vi "Open Btrfly Example.vi"() -> ()   [LabVIEW 2018]
uses:
  <vilib>/Rock Robotics/WPI/ThirdParty/Phoenix-LabVIEW/Motor Controller/Controls/CTRE_Phoenix_MotorControl_NeutralMode.ctl
  <vilib>/Rock Robotics/WPI/ThirdParty/REV Robotics/SPARK MAX/Typedef/Spark MAX Idle Mode.ctl
  <vilib>/Rock Robotics/WPI/SafetyOutput/WPI_SafetyOutputConfigMenu.ctl
  <vilib>/Rock Robotics/WPI/RobotDrive/WPI_RobotDriveOpen2MotorWithExistingMotors.vi
panel:
  in  "Error code":bool
  in  "Neutral Mode":enum16{"Coast", "Brake"}(ring)
  in  "secondsFromNeutralToFull":dbl format="%#_13g"
  in  "Cluster":T1
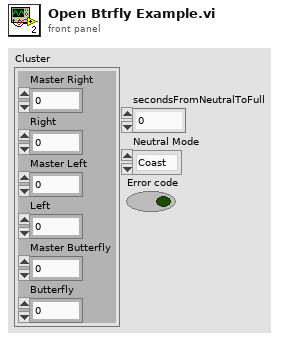
[diagram p1: front panel]
types:
  T1 = cluster{"Master Right":u8, "Right":u8, "Master Left":u8, "Left":u8, "Master Butterfly":u8, "Butterfly":u8}
  T2 = typedef "WPI_SafetyOutputConfigMenu.ctl" = enum16{"Enable", "Disable"}
  T3 = typedef "CTRE_Phoenix_MotorControl_NeutralMode.ctl" = enum8{"EEPROMSetting", "Override to Coast", "Override to Brake"}
  T4 = typedef "Spark MAX Idle Mode.ctl" = enum16{"Coast", "Brake"}
  T5 = typedef "WPI_MotorControlDeviceRef.ctl" = cluster{"DeviceStatus":errorcluster, "Type":T6, "PWM":cluster{"PWM Channel":T7, "DeadBand":T8}, "CAN":cluster{"Device Number":u8, "SetOutput VI Ref":variant, "GetOutput VI Ref":variant, "Enable VI Ref":variant, "Disable VI Ref":variant, "Data":variant}, "Invert":bool, "DIO PWM":cluster{"PWM \"Enable\" Channel":T7, "DIOChannel":T9, "PWM Rate":dbl}}
  T6 = typedef "WPI_MotorControlType.ctl" = enum16{"PWM", "CAN", "DIO PWM"}
  T7 = typedef "FPGA_DIOPWMChannel.ctl" = enum8{"PWM 0", "PWM 1", "PWM 2", "PWM 3", "PWM 4", "PWM 5", "PWM 6", "PWM 7", "PWM 8", "PWM 9", "PWM MXP 0", "PWM MXP 1", "PWM MXP 2", "PWM MXP 3", "PWM MXP 4", "PWM MXP 5", "PWM MXP 6", "PWM MXP 7", "PWM MXP 8", "PWM MXP 9", "Invalid"}
  T8 = typedef "WPI_PWMDeadband.ctl" = cluster{"Name":string, "maxPositivePwm":i32, "minPositivePwm":i32, "centerPwm":i32, "maxNegativePwm":i32, "minNegativePwm":i32, "angularRange":u16}
  T9 = typedef "FPGA_DIOChannel.ctl" = enum8{"DIO 0", "DIO 1", "DIO 2", "DIO 3", "DIO 4", "DIO 5", "DIO 6", "DIO 7", "DIO 8", "DIO 9", "DIO MXP 0", "DIO MXP 1", "DIO MXP 2", "DIO MXP 3", "DIO MXP 4", "DIO MXP 5", "DIO MXP 6", "DIO MXP 7", "DIO MXP 8", "DIO MXP 9", "DIO MXP 10", "DIO MXP 11", "DIO MXP 12", "DIO MXP 13", "DIO MXP 14", "DIO MXP 15", "SPI Port CS1", "SPI Port CS2", "SPI Port CS3", "SPI Port MISO", "SPI Port MOSI", "Invalid"}
  T10 = typedef "WPI_RobotDriveDevRef.ctl" = cluster{"DevStatus":errorcluster, "Motors[]":T5[], "Square Inputs":bool, "Max Output":dbl}
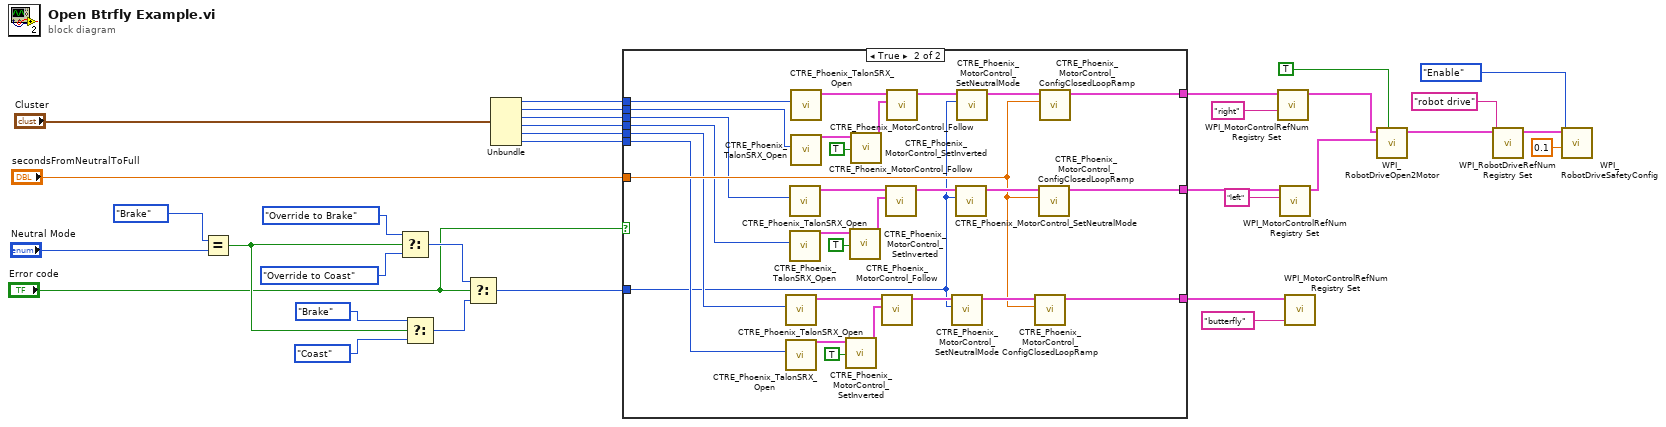
[diagram p0: block diagram]
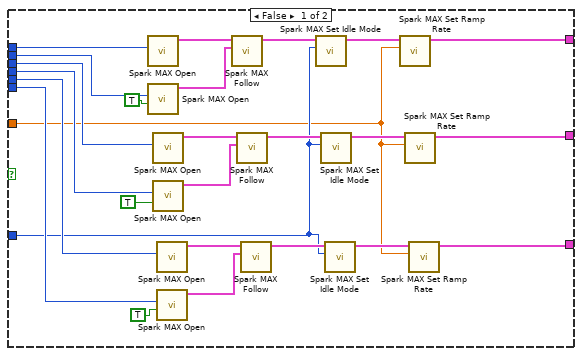
[diagram p2: hidden frame]
diagram:
  n1 = Equal?(x=enum16{"Coast", "Brake"}."Brake", y="Neutral Mode") -> (x = y?=w20:bool)
  n2 = Select(t=CTRE_Phoenix_MotorControl_NeutralMode."Override to Brake" ("Motor Control Neutral Mode"), s=w20, f=CTRE_Phoenix_MotorControl_NeutralMode."Override to Coast" ("Motor Control Neutral Mode")) -> (s? t:f=w21:T3)
  n3 = Select(t=Spark_MAX_Idle_Mode."Brake" ("Idle Mode"), s=w20, f=Spark_MAX_Idle_Mode."Coast" ("Idle Mode")) -> (s? t:f=w17:T4)
  n4 = Select(t=w21, s="Error code", f=w17) -> (s? t:f=w16:u16)
  n5 = Unbundle("Cluster") -> ("Master Right"=w31:u8, "Right"=w30:u8, "Master Left"=w29:u8, "Left"=w28:u8, "Master Butterfly"=w27:u8, "Butterfly"=w26:u8)
  n6 = case shown="True" "Error code" {
    tunnel: "secondsFromNeutralToFull" -> [w37 w70]
    tunnel: w31 -> [w46 w69]
    tunnel: w30 -> [w45 w68]
    tunnel: w29 -> [w44 w67]
    tunnel: w28 -> [w43 w66]
    tunnel: w27 -> [w42 w65]
    tunnel: w26 -> [w39 w64]
    tunnel: w16 -> [w38 w63]
    tunnel: [w36 w62] -> w14
    tunnel: [w35 w61] -> w13
    tunnel: [w34 w60] -> w12
    frame False {
      n7 = call <vilib>:"Spark MAX Open.vi"("Device Number"=w46) -> ("MotorControlDeviceRef"=w56:T5)  [unwired: 9 in, 1 out]
      n8 = call <vilib>:"Spark MAX Open.vi"("Invert"=TRUE, "Device Number"=w45) -> ("MotorControlDeviceRef"=w57:T5)  [unwired: 8 in, 1 out]
      n9 = call <vilib>:"Spark MAX Open.vi"("Device Number"=w44) -> ("MotorControlDeviceRef"=w54:T5)  [unwired: 9 in, 1 out]
      n10 = call <vilib>:"Spark MAX Open.vi"("Invert"=TRUE, "Device Number"=w43) -> ("MotorControlDeviceRef"=w53:T5)  [unwired: 8 in, 1 out]
      n11 = call <vilib>:"Spark MAX Open.vi"("Device Number"=w42) -> ("MotorControlDeviceRef"=w47:T5)  [unwired: 9 in, 1 out]
      n12 = call <vilib>:"Spark MAX Open.vi"("Invert"=TRUE, "Device Number"=w39) -> ("MotorControlDeviceRef"=w48:T5)  [unwired: 8 in, 1 out]
      n13 = call <vilib>:"Spark MAX Follow.vi"("Master Controller"=w57, "MotorControlDeviceRef"=w56) -> ("MotorControlDeviceRef"=w58:T5)  [unwired: 8 in, 1 out]
      n14 = call <vilib>:"Spark MAX Follow.vi"("Master Controller"=w53, "MotorControlDeviceRef"=w54) -> ("MotorControlDeviceRef"=w52:T5)  [unwired: 8 in, 1 out]
      n15 = call <vilib>:"Spark MAX Follow.vi"("Master Controller"=w48, "MotorControlDeviceRef"=w47) -> ("MotorControlDeviceRef"=w49:T5)  [unwired: 8 in, 1 out]
      n16 = call <vilib>:"Spark MAX Set Idle Mode.vi"("Idle Mode"=w38, "MotorControlDeviceRef in"=w58) -> ("MotorControlDeviceRef out"=w59:T5)  [unwired: 8 in, 1 out]
      n17 = call <vilib>:"Spark MAX Set Idle Mode.vi"("Idle Mode"=w38, "MotorControlDeviceRef in"=w52) -> ("MotorControlDeviceRef out"=w51:T5)  [unwired: 8 in, 1 out]
      n18 = call <vilib>:"Spark MAX Set Idle Mode.vi"("Idle Mode"=w38, "MotorControlDeviceRef in"=w49) -> ("MotorControlDeviceRef out"=w50:T5)  [unwired: 8 in, 1 out]
      n19 = call <vilib>:"Spark MAX Set Ramp Rate.vi"("Seconds from neutral to full (0)"=w37, "MotorControlDeviceRef in"=w59) -> ("MotorControlDeviceRef"=w36:T5)  [unwired: 8 in, 1 out]
      n20 = call <vilib>:"Spark MAX Set Ramp Rate.vi"("Seconds from neutral to full (0)"=w37, "MotorControlDeviceRef in"=w51) -> ("MotorControlDeviceRef"=w35:T5)  [unwired: 8 in, 1 out]
      n21 = call <vilib>:"Spark MAX Set Ramp Rate.vi"("Seconds from neutral to full (0)"=w37, "MotorControlDeviceRef in"=w50) -> ("MotorControlDeviceRef"=w34:T5)  [unwired: 8 in, 1 out]
    }
    frame True {
      n22 = call <vilib>:"CTRE_Phoenix_TalonSRX_Open.vi"("Device Number"=w65) -> ("CAN Talon SRX Ref"=w76:T5)  [unwired: 9 in, 1 out]
      n23 = call <vilib>:"CTRE_Phoenix_TalonSRX_Open.vi"("Device Number"=w64) -> ("CAN Talon SRX Ref"=w75:T5)  [unwired: 9 in, 1 out]
      n24 = call <vilib>:"CTRE_Phoenix_TalonSRX_Open.vi"("Device Number"=w67) -> ("CAN Talon SRX Ref"=w77:T5)  [unwired: 9 in, 1 out]
      n25 = call <vilib>:"CTRE_Phoenix_TalonSRX_Open.vi"("Device Number"=w66) -> ("CAN Talon SRX Ref"=w78:T5)  [unwired: 9 in, 1 out]
      n26 = call <vilib>:"CTRE_Phoenix_TalonSRX_Open.vi"("Device Number"=w69) -> ("CAN Talon SRX Ref"=w88:T5)  [unwired: 9 in, 1 out]
      n27 = call <vilib>:"CTRE_Phoenix_TalonSRX_Open.vi"("Device Number"=w68) -> ("CAN Talon SRX Ref"=w87:T5)  [unwired: 9 in, 1 out]
      n28 = call <vilib>:"CTRE_Phoenix_MotorControl_SetInverted.vi"("Invert?"=TRUE, "PhoenixMotorControlDevRef"=w75) -> ("PhoenixMotorControlDevRef"=w74:T5)  [unwired: 8 in, 1 out]
      n29 = call <vilib>:"CTRE_Phoenix_MotorControl_SetInverted.vi"("Invert?"=TRUE, "PhoenixMotorControlDevRef"=w78) -> ("PhoenixMotorControlDevRef"=w79:T5)  [unwired: 8 in, 1 out]
      n30 = call <vilib>:"CTRE_Phoenix_MotorControl_SetInverted.vi"("Invert?"=TRUE, "PhoenixMotorControlDevRef"=w87) -> ("PhoenixMotorControlDevRef"=w86:T5)  [unwired: 8 in, 1 out]
      n31 = call <vilib>:"CTRE_Phoenix_MotorControl_Follow.vi"("Master Controller to Follow"=w74, "PhoenixMotorControlDevRef"=w76) -> ("PhoenixMotorControlDevRef"=w72:T5)  [unwired: 8 in, 1 out]
      n32 = call <vilib>:"CTRE_Phoenix_MotorControl_Follow.vi"("Master Controller to Follow"=w79, "PhoenixMotorControlDevRef"=w77) -> ("PhoenixMotorControlDevRef"=w81:T5)  [unwired: 8 in, 1 out]
      n33 = call <vilib>:"CTRE_Phoenix_MotorControl_Follow.vi"("Master Controller to Follow"=w86, "PhoenixMotorControlDevRef"=w88) -> ("PhoenixMotorControlDevRef"=w84:T5)  [unwired: 8 in, 1 out]
      n34 = call <vilib>:"CTRE_Phoenix_MotorControl_SetNeutralMode.vi"("Motor Control Neutral Mode"=w63, "PhoenixMotorControlDevRef"=w72) -> ("PhoenixMotorControlDevRef"=w71:T5)  [unwired: 8 in, 1 out]
      n35 = call <vilib>:"CTRE_Phoenix_MotorControl_SetNeutralMode.vi"("Motor Control Neutral Mode"=w63, "PhoenixMotorControlDevRef"=w81) -> ("PhoenixMotorControlDevRef"=w82:T5)  [unwired: 8 in, 1 out]
      n36 = call <vilib>:"CTRE_Phoenix_MotorControl_SetNeutralMode.vi"("Motor Control Neutral Mode"=w63, "PhoenixMotorControlDevRef"=w84) -> ("PhoenixMotorControlDevRef"=w83:T5)  [unwired: 8 in, 1 out]
      n37 = call <vilib>:"CTRE_Phoenix_MotorControl_ConfigClosedLoopRamp.vi"("secondsFromNeutralToFull"=w70, "PhoenixMotorControlDevRef"=w71) -> ("PhoenixMotorControlDevRef"=w60:T5)  [unwired: 8 in, 1 out]
      n38 = call <vilib>:"CTRE_Phoenix_MotorControl_ConfigClosedLoopRamp.vi"("secondsFromNeutralToFull"=w70, "PhoenixMotorControlDevRef"=w82) -> ("PhoenixMotorControlDevRef"=w61:T5)  [unwired: 8 in, 1 out]
      n39 = call <vilib>:"CTRE_Phoenix_MotorControl_ConfigClosedLoopRamp.vi"("secondsFromNeutralToFull"=w70, "PhoenixMotorControlDevRef"=w83) -> ("PhoenixMotorControlDevRef"=w62:T5)  [unwired: 8 in, 1 out]
    }
  }
  n40 = call <vilib>:"WPI_MotorControlRefNum Registry Set.vi"("refnum name"="right", "MotorControlDevRef"=w14) -> ("MotorControlDevRef"=w8:T5)  [unwired: 8 in, 1 out]
  n41 = call <vilib>:"WPI_MotorControlRefNum Registry Set.vi"("refnum name"="left", "MotorControlDevRef"=w13) -> ("MotorControlDevRef"=w7:T5)  [unwired: 8 in, 1 out]
  n42 = call <vilib>:"WPI_MotorControlRefNum Registry Set.vi"("refnum name"="butterfly", "MotorControlDevRef"=w12) -> ()  [unwired: 8 in, 2 out]
  n43 = call-poly <vilib>:"WPI_RobotDriveOpen2Motor.vi"("Square Inputs"=TRUE, "Right Motor Dev Ref"=w7, "Left Motor Dev Ref"=w8) -> ("RobotDriveDevRef"=w5:T10)  [unwired: 7 in, 1 out]
  n44 = call <vilib>:"WPI_RobotDriveRefNum Registry Set.vi"("refnum name"="robot drive", "RobotDriveDevRef"=w5) -> ("RobotDriveDevRef"=w3:T10)  [unwired: 8 in, 1 out]
  n45 = call <vilib>:"WPI_RobotDriveSafetyConfig.vi"("timeout (s)"=0.1, "mode"=WPI_SafetyOutputConfigMenu."Enable", "RobotDriveDevRef"=w3) -> ()  [unwired: 7 in, 2 out]
